vi "Multiplier Command Insertion.vi"(6 "Opt: Timeout":u8=100, 7 "Counter Descriminator":u8, 8 "Input B":fxp<+/-,18,1>, 9 "Input A":fxp<+/-,18,1>, 10 "Channel Identifier":u8, 11 "FIFO":refnum<k21>="Multiplier 1 FIFO In :  [8b Idendifier; 20b args; 18b fxp ; 18b fxp]") -> (0 "Timeout":bool)   [LabVIEW 2009]
uses:
  <vilib>/Platform/TimedLoop/XDataNode/XDataNode.xnode
  <vilib>/Platform/TimedLoop/XDataNode/loadlvalarms.vi
  <vilib>/Platform/TimedLoop/XDataNode/timing_clust.ctl
  <vilib>/Platform/TimedLoop/XDataNode/nitl_modes.ctl
  <vilib>/Platform/TimedLoop/XDataNode/wakeup.ctl
  <vilib>/rvi/DataTransferAndStorage/Container/XNode/niFpgaContainer.xnode
  <vilib>/rvi/DataTransferAndStorage/Container/Common/niFpgaContainerMethod.ctl
  <vilib>/rvi/DataTransferAndStorage/Container/Common/niFpgaContainerExecOnDevCompGetState.vi
  <vilib>/rvi/DataTransferAndStorage/Container/Common/niFpgaContainerMetaDataKey.ctl
  <vilib>/rvi/FIFO/Fifo_Resource/nirvififoUniquifyingName.vi
  <vilib>/rvi/interface/RandomDataEmulation/niFpgaRandomDataHandleErrors.vi
  <vilib>/rvi/interface/RandomDataEmulation/nirviRandomDataFPGAFIFO.vi
  <vilib>/rvi/DataTransferAndStorage/Container/Common/niFpgaTransferTypeControl.ctl
  <vilib>/rvi/DataTransferAndStorage/FIFO/niFpgaPeerToPeerStreamState.ctl
  <vilib>/rvi/eio/common/nirviEmuReportErrorAndStop.vi
  Motor Control Global.vi
  <vilib>/Platform/TimedLoop/XDataNode/XDNodeRunTimeDep.lvlib
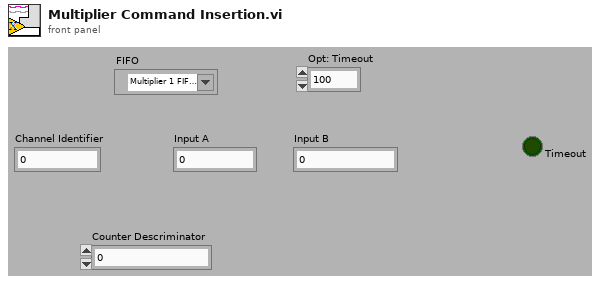
[diagram p1: front panel]
types:
  T1 = typedef "niFpgaContainerMethod.ctl" = enum16{"Write", "Read", "Clear", "Get Number of Elements to Write", "Get Number of Elements to Read", "Enable", "Disable", "Flush and Disable", "Get Stream State"}
  T2 = typedef "niFpgaTransferTypeControl.ctl" = enum16{"Target-Scoped", "Host to Target - DMA", "Target to Host - DMA", "Peer to Peer Reader", "Peer to Peer Writer", "Bidirectional"}
  T3 = typedef "niFpgaPeerToPeerStreamState.ctl" = enum16{"Unlinked", "Disabled", "Enabled", "Flushing"}
  T4 = typedef "niFpgaContainerMetaDataKey.ctl" = enum16{"FPGA FIFO", "FPGA Memory", "FPGA Register"}
  T5 = typedef "XDNodeRunTimeDep.lvlib/timing_clust.ctl" = cluster{"Expected End [f-1]":u64, "Actual End [f-1]":u64, "Finished Late? [f-1]":bool, "Expected End [i-1]":u64, "Actual End [i-1]":u64, "Finished Late? [i-1]":bool, "Expected Start [i]":u64, "Actual Start [i]":u64, "Expected Start [f]":u64, "Actual Start [f]":u64, "Source Name":string, "Structure Name":string, "Period":i64, "Deadline":i64, "Offset":i64, "Start":i64, "Priority":i32, "Timeout":i32, "Mode":T6, "Wakeup Reason":T7, "Error":errorcluster, "Source Type":string, "Secondary Source Type":string, "Global End Time":u64, "Global Start Time":u64, "Frame Duration":u64, "Iteration Duration":u64, "Assigned CPU":i32, "I/O Scan Engine Mode":u32}
  T6 = typedef "XDNodeRunTimeDep.lvlib/nitl_modes.ctl" = enum32{"No Change", "Process missed periods, maintain original phase", "Discard missed periods, maintain original phase", "Process missed periods, ignore original phase", "Discard missed periods, ignore original phase"}
  T7 = typedef "XDNodeRunTimeDep.lvlib/wakeup.ctl" = enum32{"Normal", "Aborted", "Asynchronous wakeup", "Timing source error", "Timed loop error", "Timeout"}
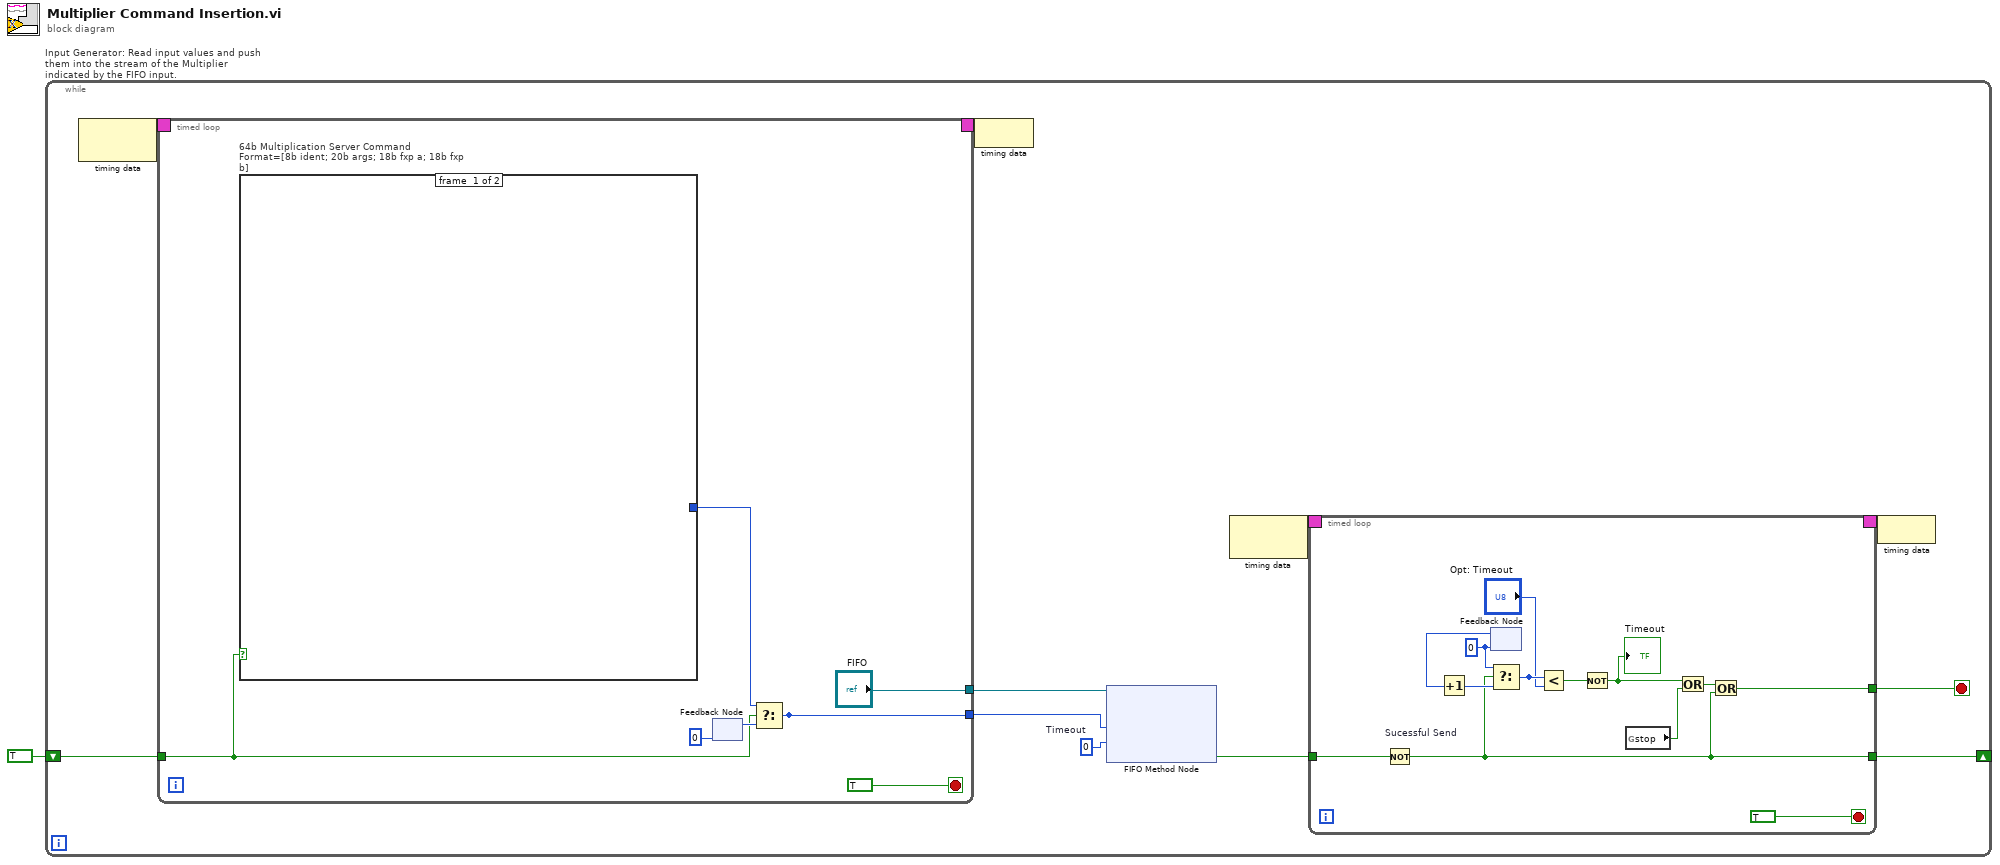
[diagram p0: block diagram]
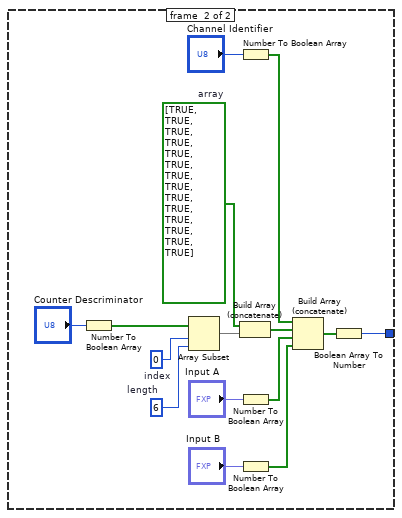
[diagram p2: hidden frame]
diagram:
  n1 = while "Input Generator: Read input values and push them into the stream of the Multiplier indicated by the FIFO input." {
    shift-right: [w8] -> _
    shift-left: TRUE -> [w11]
    stop <- w9 stop-if-true
    w4 = 0  # Timeout
    n2 = node-c288() -> (w6:T5)  [unwired: 1 in]
    n3 = timed-loop {
      timing: w6 -> [_]
      timing-out: [_] -> w5
      tunnel: w11 -> [w34]
      tunnel: ["FIFO"] -> w10
      tunnel: [w31] -> w7
      stop <- TRUE stop-if-true
      n4 = case "64b Multiplication Server Command Format=[8b ident; 20b args; 18b fxp a; 18b fxp b]" shown="True" w34 {
        tunnel: [_ w47] -> w36
        frame #0 {
        }
        frame #1 {
          w40 = bool[] [TRUE, TRUE, TRUE, TRUE, TRUE, TRUE, TRUE, TRUE, TRUE, TRUE, TRUE, TRUE, TRUE, TRUE]  # array
          w41 = 6  # length
          w42 = 0  # index
          n5 = Number To Boolean Array(number="Counter Descriminator") -> (Boolean array=w43:bool[])
          n6 = Array Subset(array=w43, index=w42, length=w41) -> (w39:bool[])
          n7 = Build Array (concatenate)(w40, w39) -> (w38:bool[])
          n8 = Number To Boolean Array(number="Channel Identifier") -> (Boolean array=w50:bool[])
          n9 = Number To Boolean Array(number="Input A") -> (Boolean array=w49:bool[])
          n10 = Number To Boolean Array(number="Input B") -> (Boolean array=w48:bool[])
          n11 = Build Array (concatenate)(w50, w38, w49, w48) -> (w37:bool[])
          n12 = Boolean Array To Number(Boolean array=w37) -> (number=w47:u64)
        }
      }
      n13 = feedback #1(u64 0) -> (w35:u64)
      n14 = Select(t=w36, s=w34, f=w35) -> (s? t:f=w31:u64)
    }
    n15 = node-c288(w5) -> ()
    n16 = xnode ("FIFO Method Node")("Element"=w7, "Timeout"=w4, "FIFO In"=w10) -> ("Timed Out?"=w12:bool)  [unwired: 1 out]
    n17 = node-c288() -> (w3:T5)  [unwired: 1 in]
    n18 = timed-loop {
      timing: w3 -> [_]
      timing-out: [_] -> w2
      tunnel: w12 -> [w25]
      tunnel: [w15] -> w9
      tunnel: [w14] -> w8
      stop <- TRUE stop-if-true
      w23 = u8 0
      n19 = Not "Sucessful Send"(x=w25) -> (.not. x?=w14:bool)
      n20 = feedback #2(w23) -> (w24:u8)
      n21 = Increment(x=w24) -> (x+1=w22:u8)
      n22 = Select(t=w23, s=w14, f=w22) -> (s? t:f=w21:u8)
      n23 = Less?(x=w21, y="Opt: Timeout") -> (x < y?=w19:bool)
      n24 = Not(x=w19) -> (.not. x?=w16:bool)
      "Timeout" <- w16
      n25 = global read "Motor Control Global.vi" "stop"() -> (w18:bool)
      n26 = Or(x=w16, y=w18) -> (x .or. y?=w17:bool)
      n27 = Or(x=w17, y=w14) -> (x .or. y?=w15:bool)
    }
    n28 = node-c288(w2) -> ()
  }
